vi "Build Preview Map.vi"(8 "error in (no error)":errorcluster, 11 "Map Model in":refnum<class "Map Model.lvclass">) -> (0 "error out":errorcluster, 3 "Map Model out":refnum<class "Map Model.lvclass">)   [LabVIEW 2020, in "Map Model.lvlib" / "Map Model.lvclass"]
uses:
  Map Model.lvclass
  Map Model.lvclass/Map Model.ctl
  <vilib>/picture/picture.llb/Draw 4-Bit Pixmap.vi
panel:
  # "NOTICE -- YOU MUST LEAVE THIS NOTICE IN PLACE.\n\nCopyright (c) 2017, LIANG LIU Shawn.Liu.cn@gmail.com\nAll rights reserved.\n\nRedistribution and use in source and binary forms, with or without modification, are permitted provided that the following conditions are met:\n-Redistributions of source code must retain the above copyright notice, this list of conditions and the following disclaimer.\n-Redistributions in binary form must reproduce the above copyright notice, this list of conditions and the following disclaimer in the documentation and/or other materials provided with the distribution.\n-Neither the name of the eLp nor the names of its contributors may be used to endorse or promote products derived from this software without specific prior written permission.\n\nTHIS SOFTWARE IS PROVIDED BY THE COPYRIGHT HOLDERS AND CONTRIBUTORS \"AS IS\" AND ANY EXPRESS OR IMPLIED WARRANTIES, INCLUDING, BUT NOT LIMITED TO, THE IMPLIED WARRANTIES OF MERCHANTABILITY AND FITNESS FOR A PARTICULAR PURPOSE ARE DISCLAIMED. IN NO EVENT SHALL THE COPYRIGHT HOLDER OR CONTRIBUTORS BE LIABLE FOR ANY DIRECT, INDIRECT, INCIDENTAL, SPECIAL, EXEMPLARY, OR CONSEQUENTIAL DAMAGES (INCLUDING, BUT NOT LIMITED TO, PROCUREMENT OF SUBSTITUTE GOODS OR SERVICES; LOSS OF USE, DATA, OR PROFITS; OR BUSINESS INTERRUPTION) HOWEVER CAUSED AND ON ANY THEORY OF LIABILITY, WHETHER IN CONTRACT, STRICT LIABILITY, OR TORT (INCLUDING NEGLIGENCE OR OTHERWISE) ARISING IN ANY WAY OUT OF THE USE OF THIS SOFTWARE, EVEN IF ADVISED OF THE POSSIBILITY OF SUCH DAMAGE."
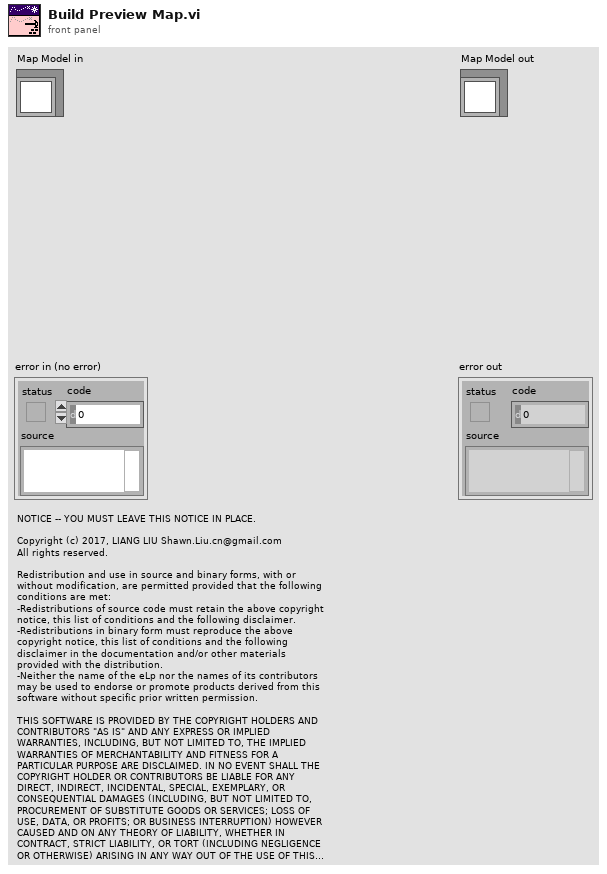
[diagram p1: front panel]
types:
  T1 = cluster{"Occupied Color":cluster{"Value":u8, "Color":u32}, "Free Color":cluster{"Value":u8, "Color":u32}, "Unknown Color":cluster{"Value":u8, "Color":u32}}
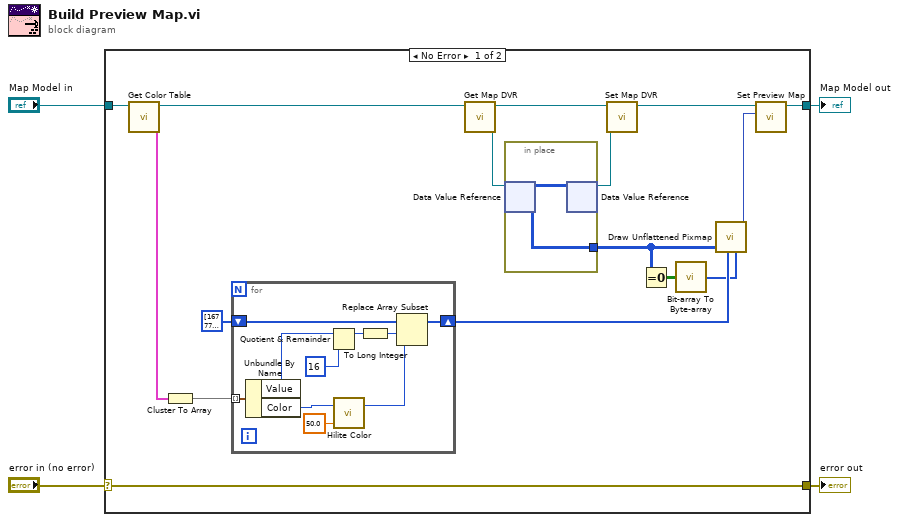
[diagram p0: block diagram]
diagram:
  n1 = case shown="No Error" "error in (no error)" {
    selector: "error in (no error)" -> [w18 w33]
    tunnel: "Map Model in" -> [w20 w32]
    tunnel: [w19 w32] -> w3
    tunnel: [w18 w33] -> w1
    frame No Error {
      n2 = call "Get Color Table.vi"("Map Model in"=w20) -> ("Color Table"=w13:T1, "Map Model out"=w11:refnum<class "Map Model.lvclass">)  [unwired: 9 in]
      n3 = Cluster To Array(cluster=w13) -> (array=w12:cluster{"Value":u8, "Color":u32}[])
      n4 = for {
        shift-right: [w29] -> w10
        shift-left: u32[] [16777215, 16776960, 128, 16711680, 16711935, 8388736, 255, 65535, 65280, 32768, 8388608, 8421376, 12632256, 8421504, 32896, 0] ("color table") -> [w30]
        tunnel: w12 -> [w28] mode=indexing
        n5 = Unbundle By Name(w28) -> ("Value"=w27:u8, "Color"=w25:u32)
        n6 = Quotient & Remainder(x=w27, y=u8 16) -> (x-y*floor(x/y)=w26:u8)  [unwired: 1 out]
        n7 = call <vilib>:"Hilite Color.vi"("Percentage(30)"=50.0, "Color In"=w25) -> ("Hilite"=w22:u32)  [unwired: 1 out]
        n8 = To Long Integer(number=w26) -> (32bit integer=w24:i32)
        n9 = Replace Array Subset(array=w30, new element=w22, index=w24) -> (w29:u32[])
      }
      n10 = call "Get Map DVR.vi"("Map Model in"=w11) -> ("Map DVR"=w15:refnum<data-value>, "Map Model out"=w17:refnum<class "Map Model.lvclass">)  [unwired: 9 in]
      n11 = in-place {
        in-place-border: [w31] -> w6
        n12 = in-place-dvr #1(w15) -> (w31:u8[][])  [unwired: 1 out]
        n13 = in-place-dvr #1(w31) -> (w16:refnum<data-value>)  [unwired: 1 out]
      }
      n14 = call "Set Map DVR.vi"("Map DVR"=w16, "Map Model in"=w17) -> ("Map Model out"=w9:refnum<class "Map Model.lvclass">)  [unwired: 9 in]
      n15 = Equal To 0?(x=w6) -> (x = 0?=w8:bool[][])
      n16 = call <vilib>:"Bit-array To Byte-array.vi"("bit array"=w8) -> ("byte array"=w7:u8[])
      n17 = call-poly <vilib>:"Draw Unflattened Pixmap.vi"("data"=w6, "color table"=w10, "mask"=w7) -> ("new picture"=w5:picture)  [unwired: 6 in]
      n18 = call "Set Preview Map.vi"("Preview Map"=w5, "Map Model in"=w9) -> ("Map Model out"=w19:refnum<class "Map Model.lvclass">)  [unwired: 9 in]
    }
    frame Error {
    }
  }
  "error out" <- w1
  "Map Model out" <- w3
